vi "observacao.vi"() -> ()   [LabVIEW 2018, in "Shared_160.lvlib"] (continued)
                w2479 = u16 15 items=["Alarme", "Atencao", "Erro", "Ocupado", "PosSecund", "PosConj#3", "MovFoco", "MovCjto#3", "Mov#4", "Mov#3", "Mov#2", "EspLamp", "HE", "NE", "EspLampRepouso", "EspLampCalibra"] ("NomeStatus")
                w2480 = u16 14 items=["Alarme", "Atencao", "Erro", "Ocupado", "PosSecund", "PosConj#3", "MovFoco", "MovCjto#3", "Mov#4", "Mov#3", "Mov#2", "EspLamp", "HE", "NE", "EspLampRepouso", "EspLampCalibra"] ("NomeStatus")
                w2481 = u16 11 items=["Alarme", "Atencao", "Erro", "Ocupado", "PosSecund", "PosConj#3", "MovFoco", "MovCjto#3", "Mov#4", "Mov#3", "Mov#2", "EspLamp", "HE", "NE", "EspLampRepouso", "EspLampCalibra"] ("NomeStatus")
                # "Cassegrain"
                n1920 = event shown="[3] \"Sent_EspLampCass\": Value Change" {
                  selector: _ -> [_ _ _ _]
                  dyn-events: _ -> [_ _ _ _]
                  timeout: 10 -> [_ _ _ _]
                  event Timeout {
                    n1921 = event-data() -> ()  [unwired: 1 in, 2 out]
                  }
                  event "Ne": Value Change {
                    w2508 = u16 3 items=["ZERO", "AH", "DEC", "TUBO", "CUP"] ("Controlador")
                    n1922 = event-data() -> ()  [unwired: 1 in, 1 out]
                    n1923 = case shown="True" "Ne" {
                      tunnel: ["LAMP_NE" "LAMP_NE"] -> w2507
                      tunnel: ["DESLIGAR" "LIGAR"] -> w2506
                      frame False {
                      }
                      frame True {
                      }
                    }
                    n1924 = call "Monta Comando.vi"("Comando"=w2506, "Dispositivo"=w2507, "Controlador"=w2508) -> ()  [unwired: 2 in, 5 out]
                  }
                  event "He-Ar": Value Change {
                    w2516 = u16 3 items=["ZERO", "AH", "DEC", "TUBO", "CUP"] ("Controlador")
                    n1925 = event-data() -> ()  [unwired: 1 in, 1 out]
                    n1926 = case shown="False" "He-Ar" {
                      tunnel: ["LAMP_HE" "LAMP_HE"] -> w2515
                      tunnel: ["DESLIGAR" "LIGAR"] -> w2514
                      frame False {
                      }
                      frame True {
                      }
                    }
                    n1927 = call "Monta Comando.vi"("Comando"=w2514, "Dispositivo"=w2515, "Controlador"=w2516) -> ()  [unwired: 2 in, 5 out]
                  }
                  event "Sent_EspLampCass": Value Change {
                    w2524 = u16 3 items=["ZERO", "AH", "DEC", "TUBO", "CUP"] ("Controlador")
                    n1928 = event-data() -> ()  [unwired: 1 in, 1 out]
                    n1929 = property on="SlideEcass" class="Slide (strict)"("Visible"=TRUE) -> ()  [unwired: 2 in, 2 out]
                    n1930 = case shown="False" "Sent_EspLampCass" {
                      tunnel: ["ESP_LAMP" "ESP_LAMP"] -> w2523
                      tunnel: ["RECUAR" "AVANCAR"] -> w2522
                      frame False {
                      }
                      frame True {
                      }
                    }
                    n1931 = property on="stopEcass" class="Bool"("Visible"=FALSE) -> ()  [unwired: 2 in, 2 out]
                    n1932 = call "Monta Comando.vi"("Comando"=w2522, "Dispositivo"=w2523, "Controlador"=w2524) -> ()  [unwired: 2 in, 5 out]
                    "SlideEcass" <- u8 8 ("Slide")
                  }
                }
                n1933 = call "Bit Status TUBO.vi"("NomeStatus"=w2477) -> ("StatBit"=→"LedHe":bool)
                n1934 = call "Bit Status TUBO.vi"("NomeStatus"=w2478) -> ("StatBit"=→"LedNe":bool)
                n1935 = call "Bit Status TUBO.vi"("NomeStatus"=w2481) -> ("StatBit"=w2476:bool)
                n1936 = call "Bit Status TUBO.vi"("NomeStatus"=w2480) -> ("StatBit"=w2475:bool)
                n1937 = call "Bit Status TUBO.vi"("NomeStatus"=w2479) -> ("StatBit"=w2474:bool)
                n1938 = And(x=w2476, y=w2475) -> (x .and. y?=w2473:bool)
                "LedRep" <- w2473
                n1939 = And(x=w2476, y=w2474) -> (x .and. y?=w2472:bool)
                "LedCal" <- w2472
                n1940 = property on="SlideEcass" class="Slide (strict)"() -> ("Visible"=w2471:bool)  [unwired: 2 in, 2 out]
                n1941 = Or(x=w2473, y=w2472) -> (x .or. y?=w2483:bool)
                n1942 = Or(x=w2475, y=w2474) -> (x .or. y?=w2486:bool)
                n1943 = Not(x=w2476) -> (.not. x?=w2485:bool)
                n1944 = And(x=w2471, y=w2483) -> (x .and. y?=w2482:bool)
                n1945 = And(x=w2485, y=w2486) -> (x .and. y?=w2484:bool)
                n1946 = case shown="True" "stopEcass" {
                  frame False {
                  }
                  frame True {
                    w2503 = FALSE
                    w2502 = u8 0 ("Disabled")
                    w2501 = u16 3 items=["ZERO", "AH", "DEC", "TUBO", "CUP"] ("Controlador")
                    n1947 = call "Monta Comando.vi"("Comando"="DESLIGAR", "Dispositivo"="ESP_LAMP", "Controlador"=w2501) -> ()  [unwired: 2 in, 5 out]
                    n1948 = property on="Sent_EspLampCass" class="Bool (strict)"("Disabled"=w2502) -> ()  [unwired: 2 in, 2 out]
                    n1949 = property on="Ne" class="Bool (strict)"("Disabled"=w2502) -> ()  [unwired: 2 in, 2 out]
                    n1950 = property on="He-Ar" class="Bool (strict)"("Disabled"=w2502) -> ()  [unwired: 2 in, 2 out]
                    n1951 = property on="SlideEcass" class="Slide (strict)"("Visible"=w2503) -> ()  [unwired: 2 in, 2 out]
                    n1952 = property on="stopEcass" class="Bool"("Visible"=w2503) -> ()  [unwired: 2 in, 2 out]
                  }
                }
                n1953 = case shown="True" w2482 {
                  frame False {
                  }
                  frame True {
                    w2504 = u8 0 ("Disabled")
                    n1954 = property on="Sent_EspLampCass" class="Bool (strict)"("Disabled"=w2504) -> ()  [unwired: 2 in, 2 out]
                    n1955 = property on="He-Ar" class="Bool (strict)"("Disabled"=w2504) -> ()  [unwired: 2 in, 2 out]
                    n1956 = property on="Ne" class="Bool (strict)"("Disabled"=w2504) -> ()  [unwired: 2 in, 2 out]
                    n1957 = property on="SlideEcass" class="Slide (strict)"("Visible"=FALSE) -> ()  [unwired: 2 in, 2 out]
                  }
                }
                n1958 = case shown="True" w2484 {
                  frame False {
                  }
                  frame True {
                    w2488 = u8 2 ("Disabled")
                    n1959 = local read "SlideEcass"() -> (w2489:u8)
                    n1960 = property on="Sent_EspLampCass" class="Bool (strict)"("Disabled"=w2488) -> ()  [unwired: 2 in, 2 out]
                    n1961 = property on="Ne" class="Bool (strict)"("Disabled"=w2488) -> ()  [unwired: 2 in, 2 out]
                    n1962 = property on="He-Ar" class="Bool (strict)"("Disabled"=w2488) -> ()  [unwired: 2 in, 2 out]
                    n1963 = Add(x=w2489, y=u8 4) -> (x+y=w2491:u8)
                    n1964 = Greater Or Equal?(x=w2491, y=u8 100 ("x")) -> (x >= y?=w2492:bool)
                    n1965 = case shown="True" w2492 {
                      selector: w2492 -> [_ w2496]
                      tunnel: w2491 -> [w2495 _]
                      frame False {
                        n1966 = local write "SlideEcass"(w2495) -> ()
                        n1967 = property on="SlideEcass" class="Slide (strict)"("Fill Color"=u32 16750950 ("color(black)")) -> ()  [unwired: 2 in, 2 out]
                      }
                      frame True {
                        n1968 = local write "SlideEcass"(u8 92 ("Slide")) -> ()
                        n1969 = property on="stopEcass" class="Bool"("Visible"=w2496) -> ()  [unwired: 2 in, 2 out]
                        n1970 = property on="SlideEcass" class="Slide (strict)"("Fill Color"=u32 16724787 ("color(black)")) -> ()  [unwired: 2 in, 2 out]
                      }
                    }
                  }
                }
              }
              frame "Eucalyp." {
                # "Eucalyptus"
              }
              frame "Cam 1" {
              }
              frame "Cam 2" {
                # "Cam 2"
              }
              frame "Cam IV." {
                # "Cam IV"
              }
              frame "Polarim." {
                # "Polarimetro"
              }
              frame "Fotrap" {
                # "Fotrap"
              }
              frame "Coude", Default {
                # "COUDE"
                n1971 = stacked-sequence {
                  frame #0 {
                    w2535 = u16 5 items=["Alarme", "Atencao", "Erro", "Ocupado", "Stop#3", "Cass#3", "MovFoco", "PosSecund", "Mov#2", "Mov#3", "Mov#4", "EspLamp", "HE", "NE", "EspLampRepouso", "EspLampCalibra"] ("NomeStatus")
                    w2534 = u16 7 items=["Alarme", "Atencao", "Erro", "Ocupado", "Stop#3", "Cass#3", "MovFoco", "PosSecund", "Mov#2", "Mov#3", "Mov#4", "EspLamp", "HE", "NE", "EspLampRepouso", "EspLampCalibra"] ("NomeStatus")
                    n1972 = local read "EspAtual"() -> (w2537:string)
                    n1973 = case shown="\"A\"" w2537 {
                      frame "X", Default {
                        w2538 = FALSE
                        n1974 = local write "ledVisivel"(w2538) -> ()
                        n1975 = local write "ledAzul"(w2538) -> ()
                        n1976 = local write "ledVermelho"(w2538) -> ()
                      }
                      frame "M" {
                        w2539 = FALSE
                        n1977 = local write "ledAzul"(w2539) -> ()
                        n1978 = local write "ledVermelho"(w2539) -> ()
                        n1979 = local write "ledVisivel"(w2539) -> ()
                      }
                      frame "A" {
                        # "Espelho A --> Azul\nEspelho B --> Visível\nEspelho C --> Vermelho"
                        n1980 = local write "ledVermelho"(FALSE) -> ()
                        n1981 = local write "ledVisivel"(FALSE) -> ()
                        n1982 = local write "ledAzul"(TRUE) -> ()
                      }
                      frame "B" {
                        # "Espelho A --> Azul\nEspelho B --> Visível\nEspelho C --> Vermelho"
                        n1983 = local write "ledVermelho"(FALSE) -> ()
                        n1984 = local write "ledVisivel"(TRUE) -> ()
                        n1985 = local write "ledAzul"(FALSE) -> ()
                      }
                      frame "C" {
                        # "Espelho A --> Azul\nEspelho B --> Visível\nEspelho C --> Vermelho"
                        n1986 = local write "ledVermelho"(TRUE) -> ()
                        n1987 = local write "ledVisivel"(FALSE) -> ()
                        n1988 = local write "ledAzul"(FALSE) -> ()
                      }
                    }
                    n1989 = call "Bit Status TUBO.vi"("NomeStatus"=w2535) -> ("StatBit"=→"Cjto_3":bool)
                    n1990 = call "Bit Status TUBO.vi"("NomeStatus"=w2534) -> ("StatBit"=→"PosSecundario":bool)
                  }
                  frame #1 {
                    w2559 = u16 5 items=["Alarme", "Atencao", "Erro", "Ocupado", "Stop#3", "Cass#3", "MovFoco", "PosSecund", "Mov#2", "Mov#3", "Mov#4", "EspLamp", "HE", "NE", "EspLampRepouso", "EspLampCalibra"] ("NomeStatus")
                    w2564 = u16 8 items=["Alarme", "Atencao", "Erro", "Ocupado", "Stop#3", "Cass#3", "MovFoco", "PosSecund", "Mov#2", "Mov#3", "Mov#4", "EspLamp", "HE", "NE", "EspLampRepouso", "EspLampCalibra"] ("NomeStatus")
                    w2565 = u16 9 items=["Alarme", "Atencao", "Erro", "Ocupado", "Stop#3", "Cass#3", "MovFoco", "PosSecund", "Mov#2", "Mov#3", "Mov#4", "EspLamp", "HE", "NE", "EspLampRepouso", "EspLampCalibra"] ("NomeStatus")
                    w2566 = u16 10 items=["Alarme", "Atencao", "Erro", "Ocupado", "Stop#3", "Cass#3", "MovFoco", "PosSecund", "Mov#2", "Mov#3", "Mov#4", "EspLamp", "HE", "NE", "EspLampRepouso", "EspLampCalibra"] ("NomeStatus")
                    w2577 = u16 4 items=["Alarme", "Atencao", "Erro", "Ocupado", "Stop#3", "Cass#3", "MovFoco", "PosSecund", "Mov#2", "Mov#3", "Mov#4", "EspLamp", "HE", "NE", "EspLampRepouso", "EspLampCalibra"] ("NomeStatus")
                    w2578 = u16 3 items=["Alarme", "Atencao", "Erro", "Ocupado", "Stop#3", "Cass#3", "MovFoco", "PosSecund", "Mov#2", "Mov#3", "Mov#4", "EspLamp", "HE", "NE", "EspLampRepouso", "EspLampCalibra"] ("NomeStatus")
                    # "CJTO#3 EM \nMOVIMENTO"
                    n1991 = local read "PosSecundario"() -> (w2557:bool)
                    n1992 = call "Bit Status TUBO.vi"("NomeStatus"=w2559) -> ("StatBit"=w2556:bool)
                    n1993 = call "Bit Status TUBO.vi"("NomeStatus"=w2577) -> ("StatBit"=w2555:bool)
                    n1994 = call "Bit Status TUBO.vi"("NomeStatus"=w2578) -> ("StatBit"=w2553:bool)
                    n1995 = call "Bit Status TUBO.vi"("NomeStatus"=w2564) -> ("StatBit"=w2570:bool)
                    "#2" <- w2570
                    n1996 = call "Bit Status TUBO.vi"("NomeStatus"=w2565) -> ("StatBit"=w2569:bool)
                    "#3" <- w2569
                    n1997 = call "Bit Status TUBO.vi"("NomeStatus"=w2566) -> ("StatBit"=w2568:bool)
                    "#4" <- w2568
                    n1998 = Not Equal?(x=w2557, y=w2556) -> (x != y?=w2558:bool)
                    n1999 = Not(x=w2555) -> (.not. x?=w2551:bool)
                    n2000 = And(x=w2558, y=w2555) -> (x .and. y?=w2552:bool)
                    n2001 = Compound Arithmetic op=OR(w2570, w2569, w2568) -> (w2567:bool)
                    n2002 = Compound Arithmetic op=OR(w2552, w2551, w2553) -> (w2554:bool)
                    n2003 = property on="Cjto_3" class="Bool (strict)"("Blinking"=w2552) -> ()  [unwired: 2 in, 2 out]
                    n2004 = property on="PosSecundario" class="Bool (strict)"("Blinking"=w2552) -> ()  [unwired: 2 in, 2 out]
                    n2005 = case shown="True" w2554 {
                      tunnel: [T6."Page Enabled" ("Page Enabled State") T6."Page Disabled" ("Page Enabled State")] -> w2549
                      tunnel: [u8 0 ("Disabled") u8 2 ("Disabled")] -> w2563
                      frame False {
                      }
                      frame True {
                      }
                    }
                    n2006 = property on="MENSAGEM" class="Str"("Visible"=w2551, "Blinking"=w2551) -> ()  [unwired: 2 in, 2 out]
                    n2007 = case shown="True" w2567 {
                      tunnel: w2563 -> [w2582 _]
                      tunnel: [w2582 u8 2 ("Disabled")] -> w2562
                      tunnel: [FALSE TRUE] -> w2561
                      tunnel: [FALSE ("Blinking") TRUE ("Blinking")] -> w2560
                      frame False {
                        n2008 = local write "MENSAGEM 2"("EM MOVIMENTO" ("MENSAGEM 2")) -> ()
                      }
                      frame True {
                        n2009 = local read "EndTime"() -> (w2591:u32)
                        n2010 = Tick Count (ms)() -> (millisecond timer value=w2590:u32)
                        n2011 = Subtract(x=w2591, y=w2590) -> (x-y=w2589:u32)
                        n2012 = Divide(x=w2589, y=u32 1000) -> (x/y=w2586:dbl)
                        n2013 = To Unsigned Long Integer(number=w2586) -> (unsigned 32bit integer=w2587:u32)
                        n2014 = Number To Decimal String(number=w2587) -> (decimal integer string=w2584:string)  [unwired: 1 in]
                        n2015 = Concatenate Strings("EM MOVIMENTO " ("MENSAGEM 2"), w2584) -> (w2585:string)
                        n2016 = local write "MENSAGEM 2"(w2585) -> ()
                      }
                    }
                    n2017 = property on="Setup, Pointing & Guiding" class="TabCtl (strict)"() -> ("Pages"=w2550:refnum<vi>[])  [unwired: 2 in, 2 out]
                    n2018 = Index Array(array=w2550, index=4) -> (element=w2573:refnum<vi>)
                    n2019 = Index Array(array=w2550, index=5) -> (element=w2576:refnum<vi>)
                    n2020 = property class="Page"(reference=w2573, "Page Enabled State"=w2549) -> ()  [unwired: 1 in, 2 out]
                    n2021 = property class="Page"(reference=w2576, "Page Enabled State"=w2549) -> ()  [unwired: 1 in, 2 out]
                    n2022 = case shown="False" w2557 {
                      tunnel: [u8 0 ("Disabled") w2597] -> w2572
                      tunnel: w2562 -> [w2595 _]
                      tunnel: [w2595 w2597] -> w2571
                      frame False {
                        # "COUDE"
                      }
                      frame True {
                        w2597 = u8 2 ("Disabled")
                        # "CASS"
                      }
                    }
                    n2023 = property on="MENSAGEM 2" class="Str"("Visible"=w2561, "Blinking"=w2560) -> ()  [unwired: 2 in, 2 out]
                    n2024 = property on="ledAzul" class="Bool (strict)"("Disabled"=w2572) -> ()  [unwired: 2 in, 2 out]
                    n2025 = property on="ledVisivel" class="Bool (strict)"("Disabled"=w2572) -> ()  [unwired: 2 in, 2 out]
                    n2026 = property on="ledVermelho" class="Bool (strict)"("Disabled"=w2572) -> ()  [unwired: 2 in, 2 out]
                    n2027 = property on="Radio Buttons" class="RadioBtnsControl (strict)"("Disabled"=w2572) -> ()  [unwired: 2 in, 2 out]
                    n2028 = property on="#2" class="Bool (strict)"("Disabled"=w2572) -> ()  [unwired: 2 in, 2 out]
                    n2029 = property on="#3" class="Bool (strict)"("Disabled"=w2572) -> ()  [unwired: 2 in, 2 out]
                    n2030 = property on="#4" class="Bool (strict)"("Disabled"=w2572) -> ()  [unwired: 2 in, 2 out]
                    n2031 = property on="Go_Coudé" class="Bool"("Disabled"=w2571) -> ()  [unwired: 2 in, 2 out]
                  }
                  frame #2 {
                    n2032 = case shown="True" "Go_Coudé" {
                      frame False {
                        w2603 = u16 2 items=["Alarme", "Atencao", "Erro", "Ocupado", "Stop#3", "Cass#3", "MovFoco", "PosSecund", "Mov#2", "Mov#3", "Mov#4", "EspLamp", "HE", "NE", "EspLampRepouso", "EspLampCalibra"] ("NomeStatus")
                        w2604 = u16 3 items=["Alarme", "Atencao", "Erro", "Ocupado", "Stop#3", "Cass#3", "MovFoco", "PosSecund", "Mov#2", "Mov#3", "Mov#4", "EspLamp", "HE", "NE", "EspLampRepouso", "EspLampCalibra"] ("NomeStatus")
                        # "TRATA ERROS DO CONTROLADOR"
                        n2033 = call "Bit Status TUBO.vi"("NomeStatus"=w2603) -> ("StatBit"=w2606:bool)
                        n2034 = call "Bit Status TUBO.vi"("NomeStatus"=w2604) -> ("StatBit"=w2608:bool)
                        n2035 = Not(x=w2608) -> (.not. x?=w2607:bool)
                        n2036 = And(x=w2606, y=w2607) -> (x .and. y?=w2605:bool)
                        n2037 = case shown="True" w2605 {
                          frame False {
                          }
                          frame True {
                            w2611 = u16 3 items=["ZERO", "AH", "DEC", "TUBO", "CUP"] ("Controlador")
                            n2038 = call "Monta Comando.vi"("Comando"="ERROS", "Dispositivo"="PROG" ("Comando"), "Controlador"=w2611) -> ()  [unwired: 2 in, 5 out]
                          }
                        }
                      }
                      frame True {
                        w2612 = u16 3 items=["ZERO", "AH", "DEC", "TUBO", "CUP"] ("Controlador")
                        # "Enviar comando de \nmudar Espelho ABC"
                        n2039 = local read "EspAtual"() -> (w2618:string)
                        n2040 = case shown="\"Visível\"" "Radio Buttons" {
                          tunnel: ["C" ("Comando") "A" ("Comando") "B" ("Comando")] -> w2613
                          tunnel: w2618 -> [w2621 w2627 w2632]
                          tunnel: [w2620 w2626 w2633] -> w2615
                          frame "Vermelho" {
                            n2041 = case shown="\"A\"" w2621 {
                              tunnel: [u32 0 u32 60000 u32 35000] -> w2620
                              frame "C", Default {
                              }
                              frame "B" {
                              }
                              frame "A" {
                              }
                            }
                          }
                          frame "Azul", Default {
                            n2042 = case shown="\"C\"" w2627 {
                              tunnel: [u32 0 u32 35000 u32 60000] -> w2626
                              frame "A", Default {
                              }
                              frame "B" {
                              }
                              frame "C" {
                              }
                            }
                          }
                          frame "Visível" {
                            n2043 = case shown="\"C\"" w2632 {
                              tunnel: [u32 0 u32 60000 u32 35000] -> w2633
                              frame "B", Default {
                              }
                              frame "A" {
                              }
                              frame "C" {
                              }
                            }
                          }
                        }
                        n2044 = Tick Count (ms)() -> (millisecond timer value=w2617:u32)
                        n2045 = Add(x=w2617, y=w2615) -> (x+y=→"EndTime":u32)
                        n2046 = call "Monta Comando.vi"("Comando"=w2613, "Dispositivo"="ESPELHO" ("Comando"), "Controlador"=w2612) -> ()  [unwired: 2 in, 5 out]
                      }
                    }
                  }
                  frame #3 {
                    w2644 = 360.0
                    w2649 = 6.283185307179586
                    n2047 = global read "Global_Telescopio.vi" "guide_ang"() -> (w2659:string)
                    n2048 = global read "Global_Telescopio.vi" "guide_nor"() -> (w2660:string)
                    n2049 = global read "Global_Telescopio.vi" "AH_now"() -> (w2656:dbl)
                    n2050 = global read "Global_Telescopio.vi" "delta_now"() -> (w2657:dbl)
                    n2051 = Add(x=w2656, y=w2657) -> (x+y=w2648:dbl)
                    n2052 = Fract/Exp String To Number(string=w2659) -> (number=w2655:dbl)  [unwired: 3 in, 1 out]
                    n2053 = Fract/Exp String To Number(string=w2660) -> (number=w2658:dbl)  [unwired: 3 in, 1 out]
                    n2054 = Quotient & Remainder(x=w2648, y=w2649) -> (x-y*floor(x/y)=w2651:dbl)  [unwired: 1 out]
                    n2055 = Add(x=w2655, y=w2658) -> (x+y=w2640:dbl)
                    n2056 = Less Than 0?(x=w2651) -> (x < 0?=w2653:bool)
                    n2057 = case shown="True" w2653 {
                      tunnel: w2651 -> [w2661 w2664]
                      tunnel: [w2661 w2662] -> w2650
                      tunnel: w2649 -> [_ w2663]
                      frame False {
                      }
                      frame True {
                        n2058 = Add(x=w2664, y=w2663) -> (x+y=w2662:dbl)
                      }
                    }
                    n2059 = Add(x=124.0, y=w2640) -> (x+y=w2639:dbl)
                    n2060 = Multiply(x=w2650, y=57.29577951 ("x*y")) -> (x*y=w2647:dbl)
                    n2061 = Subtract(x=98.2, y=w2647) -> (x-y=w2646:dbl)
                    n2062 = Add(x=w2639, y=w2646) -> (x+y=w2643:dbl)
                    n2063 = Quotient & Remainder(x=w2643, y=w2644) -> (floor(x/y)=w2645:dbl)  [unwired: 1 out]
                    n2064 = Multiply(x=w2645, y=w2644) -> (x*y=w2642:dbl)
                    n2065 = Subtract(x=w2643, y=w2642) -> (x-y=→"Ang. Fenda":dbl)
                  }
                  frame #4 {
                    # "90"
                    # "270"
                    # "180"
                    # "0"
                    n2066 = event shown="[7] \"Go Angulo de Difração\": Value Change" {
                      selector: _ -> [_ _ _ _ _ _ _ _ _ _ _]
                      dyn-events: _ -> [_ _ _ _ _ _ _ _ _ _ _]
                      timeout: 10 -> [_ _ _ _ _ _ _ _ _ _ _]
                      event Timeout {
                        n2067 = event-data() -> ()  [unwired: 1 in, 2 out]
                        n2068 = stacked-sequence {
                          frame #0 {
                            n2069 = local read "parou 3"() -> (w2666:bool)
                            n2070 = case shown="True" w2666 {
                              frame False {
                              }
                              frame True {
                                n2071 = call "InstrumentControl.vi"("Input Message"="COUDE REDE POSICAO") -> ("Output Message"=w2669:string)  [unwired: 9 in, 1 out]
                                "Output Message" <- w2669
                                n2072 = Decimal String To Number(string=w2669) -> (number=w2668:i32)  [unwired: 2 in, 1 out]
                                n2073 = while {
                                shift-right: [w2672] -> w2667
                                shift-left: _ -> [w2676]
                                tunnel: w2668 -> [w2672]
                                stop <- TRUE stop-if-true
                                n2074 = Subtract(x=w2676, y=w2672) -> (x-y=w2675:i32)
                                n2075 = Absolute Value(x=w2675) -> (abs(x)=w2674:i32)
                                n2076 = Greater Or Equal?(x=w2674, y=1) -> (x >= y?=→"parou 3":bool)
                                }
                                "Posição Rede" <- w2667
                              }
                            }
                          }
                          frame #1 {
                            n2077 = local read "parou"() -> (w2679:bool)
                            n2078 = local read "parou 2"() -> (w2678:bool)
                            n2079 = case shown="True" w2678 {
                              frame False {
                              }
                              frame True {
                                # "Cada volta -> 10mm\nCada volta -> 4000counts\n1 count = 0,0025mm"
                                n2080 = call "InstrumentControl.vi"("Input Message"="COUDE ESPELHO POSICAO") -> ("Output Message"=w2686:string)  [unwired: 9 in, 1 out]
                                n2081 = Fract/Exp String To Number(string=w2686) -> (number=w2685:dbl)  [unwired: 3 in, 1 out]
                                n2082 = while {
                                shift-right: [w2698] -> w2681
                                shift-left: _ -> [w2699]
                                tunnel: w2685 -> [w2698]
                                tunnel: [w2694] -> w2680
                                stop <- TRUE stop-if-true
                                n2083 = Subtract(x=w2699, y=w2698) -> (x-y=w2697:dbl)
                                n2084 = Absolute Value(x=w2697) -> (abs(x)=w2696:dbl)
                                n2085 = Greater Or Equal?(x=w2696, y=0.02) -> (x >= y?=w2694:bool)
                                "parou 2" <- w2694
                                }
                                "Posição Espelho" <- w2681
                                n2086 = case shown="False" w2680 {
                                frame False {
                                n2087 = call "InstrumentControl.vi"("Input Message"="COUDE SERIAL CHAVEAR OFF") -> ()  [unwired: 9 in, 2 out]
                                }
                                frame True {
                                }
                                }
                                n2088 = Absolute Value(x=w2681) -> (abs(x)=w2682:dbl)
                                n2089 = Less Or Equal?(x=w2682, y=0.5) -> (x <= y?=w2684:bool)
                                n2090 = case shown="False" w2684 {
                                tunnel: w2682 -> [w2691 _]
                                frame False {
                                n2091 = Greater Or Equal?(x=w2691, y=34.5) -> (x >= y?=w2689:bool)
                                n2092 = case shown="True" w2689 {
                                frame False {
                                }
                                frame True {
                                n2093 = local write "Boolean"(TRUE ("Boolean")) -> ()
                                }
                                }
                                }
                                frame True {
                                n2094 = local write "Boolean"(FALSE ("Boolean")) -> ()
                                }
                                }
                              }
                            }
                            n2095 = case shown="True" w2679 {
                              frame False {
                              }
                              frame True {
                                n2096 = call "InstrumentControl.vi"("Input Message"="COUDE FENDA POSICAO") -> ("Output Message"=w2706:string)  [unwired: 9 in, 1 out]
                                n2097 = Fract/Exp String To Number(string=w2706) -> (number=w2705:dbl)  [unwired: 3 in, 1 out]
                                n2098 = Multiply(x=w2705, y=1000.0) -> (x*y=w2703:dbl)
                                n2099 = while {
                                shift-right: [w2713] -> w2702
                                shift-left: _ -> [w2714]
                                tunnel: w2703 -> [w2713]
                                tunnel: [w2709] -> w2701
                                stop <- TRUE stop-if-true
                                n2100 = Subtract(x=w2714, y=w2713) -> (x-y=w2712:dbl)
                                n2101 = Absolute Value(x=w2712) -> (abs(x)=w2711:dbl)
                                n2102 = Greater Or Equal?(x=w2711, y=1.0) -> (x >= y?=w2709:bool)
                                "parou" <- w2709
                                }
                                "Largura da Fenda 2" <- w2702
                                n2103 = case shown="False" w2701 {
                                frame False {
                                n2104 = call "InstrumentControl.vi"("Input Message"="COUDE SERIAL CHAVEAR OFF") -> ()  [unwired: 9 in, 2 out]
                                }
                                frame True {
                                }
                                }
                              }
                            }
                          }
                        }
                      }
                      event "Cathode": Value Change {
                        n2105 = event-data() -> ("NewVal"=w2716:bool)  [unwired: 1 in, 4 out]
                        n2106 = case shown="True" w2716 {
                          frame False {
                          }
                          frame True {
                            n2107 = flat-sequence {
                              frame #0 {
                                w2718 = FALSE ("NeAr")
                                n2108 = local write "Neon"(w2718) -> ()
                                n2109 = local write "Incand"(w2718) -> ()
                                n2110 = local write "Position"("Moving" ("Prisma Position")) -> ()
                                n2111 = call "Comando_Quick_Silver.vi"("COMANDO COMPLETO"="COUDE PRISMA MOVER 0" ("Input Message")) -> ()  [unwired: 2 in, 3 out]
                                n2112 = local write "IronArc"(w2718) -> ()
                              }
                              frame #1 {
                                n2113 = Wait (ms)(milliseconds to wait=u32 50) -> ()  [unwired: 1 out]
                              }
                              frame #2 {
                                n2114 = local write "Position"("Cathode" ("Prisma Position")) -> ()
                              }
                            }
                          }
                        }
                      }
                      event "Neon": Value Change {
                        n2115 = event-data() -> ("NewVal"=w2722:bool)  [unwired: 1 in, 4 out]
                        n2116 = case shown="True" w2722 {
                          frame False {
                          }
                          frame True {
                            n2117 = flat-sequence {
                              frame #0 {
                                w2724 = FALSE ("ThAr")
                                n2118 = local write "Cathode"(w2724) -> ()
                                n2119 = local write "Incand"(w2724) -> ()
                                n2120 = local write "Position"("Moving" ("Prisma Position")) -> ()
                                n2121 = call "Comando_Quick_Silver.vi"("COMANDO COMPLETO"="COUDE PRISMA MOVER 180" ("Input Message")) -> ()  [unwired: 2 in, 3 out]
                                n2122 = local write "IronArc"(w2724) -> ()
                              }
                              frame #1 {
                                n2123 = Wait (ms)(milliseconds to wait=u32 50) -> ()  [unwired: 1 out]
                              }
                              frame #2 {
                                n2124 = local write "Position"("Neon" ("Prisma Position")) -> ()
                              }
                            }
                          }
                        }
                      }
                      event "Incand": Value Change {
                        n2125 = event-data() -> ("NewVal"=w2728:bool)  [unwired: 1 in, 4 out]
                        n2126 = case shown="True" w2728 {
                          frame False {
                          }
                          frame True {
                            n2127 = flat-sequence {
                              frame #0 {
                                w2730 = FALSE ("ThAr")
                                n2128 = local write "Cathode"(w2730) -> ()
                                n2129 = local write "Neon"(w2730) -> ()
                                n2130 = local write "Position"("Moving" ("Prisma Position")) -> ()
                                n2131 = call "Comando_Quick_Silver.vi"("COMANDO COMPLETO"="COUDE PRISMA MOVER 270 " ("Input Message")) -> ()  [unwired: 2 in, 3 out]
                                n2132 = local write "IronArc"(w2730) -> ()
                              }
                              frame #1 {
                                n2133 = Wait (ms)(milliseconds to wait=u32 50) -> ()  [unwired: 1 out]
                              }
                              frame #2 {
                                n2134 = local write "Position"("Incand" ("Prisma Position")) -> ()
                              }
                            }
                          }
                        }
                      }
                      event Value Change {
                        n2135 = event-data() -> ("NewVal"=w2734:T4)  [unwired: 1 in, 4 out]
                        n2136 = case shown="True" w2734 {
                          frame False {
                          }
                          frame True {
                            n2137 = call "InstrumentControl.vi"("Input Message"="COUDE FENDA INICIAR") -> ()  [unwired: 9 in, 2 out]
                          }
                        }
                      }
                      event Value Change {
                        n2138 = event-data() -> ("NewVal"=w2736:T4)  [unwired: 1 in, 4 out]
                        n2139 = case shown="True" w2736 {
                          frame False {
                          }
                          frame True {
                            n2140 = call "Comando_Quick_Silver.vi"("COMANDO COMPLETO"="COUDE ESPELHO INICIAR" ("Input Message")) -> ()  [unwired: 2 in, 3 out]
                          }
                        }
                      }
                      event Value Change {
                        n2141 = event-data() -> ("NewVal"=w2738:T4)  [unwired: 1 in, 4 out]
                        n2142 = case shown="True" w2738 {
                          frame False {
                          }
                          frame True {
                            n2143 = call "InstrumentControl.vi"("Input Message"="COUDE PRISMA INICIAR") -> ()  [unwired: 9 in, 2 out]
                          }
                        }
                      }
                      event "Go Angulo de Difração": Value Change {
                        n2144 = event-data() -> ("NewVal"=w2740:bool)  [unwired: 1 in, 4 out]
                        n2145 = case shown="True" w2740 {
                          frame False {
                          }
                          frame True {
                            # "Envia comando para rede de difração"
                            n2146 = Number To Decimal String(number="Angulo da rede de difração") -> (decimal integer string=w2742:string)  [unwired: 1 in]
                            n2147 = Concatenate Strings("COUDE REDE MOVER ", w2742) -> (w2745:string)
                            n2148 = call "InstrumentControl.vi"("Input Message"=w2745) -> ()  [unwired: 9 in, 2 out]
                            n2149 = local write "parou 3"(TRUE ("parou 3")) -> ()
                          }
                        }
                      }
                      event "Go Largura da Fenda": Value Change {
                        n2150 = event-data() -> ("NewVal"=w2746:bool)  [unwired: 1 in, 4 out]
                        n2151 = case shown="True" w2746 {
                          frame False {
                          }
                          frame True {
                            n2152 = call "InstrumentControl.vi"("Input Message"="COUDE SERIAL CHAVEAR ON") -> ("error out"=w2748:errorcluster)  [unwired: 9 in, 1 out]
                            n2153 = Divide(x="Largura da Fenda", y=1000.0) -> (x/y=w2756:dbl)
                            n2154 = Number To Fractional String(use system decimal point (T)=FALSE, number=w2756, precision (6)=i16 6) -> (F-format string=w2750:string)  [unwired: 1 in]
                            n2155 = Concatenate Strings("COUDE FENDA MOVER ", w2750) -> (w2752:string)
                            n2156 = local write "parou"(TRUE ("parou")) -> ()
                            n2157 = call "InstrumentControl.vi"("error"=w2748, "Input Message"=w2752) -> ()  [unwired: 8 in, 2 out]
                          }
                        }
                      }
                      event "Prisma das Lâmpadas": Value Change {
                        n2158 = event-data() -> ("NewVal"=w2767:bool)  [unwired: 1 in, 4 out]
                        n2159 = case shown="False" w2767 {
                          tunnel: [0.0 ("y") 35.0 ("y")] -> w2765
                          frame False {
                            n2160 = local write "Boolean"(TRUE ("Boolean")) -> ()
                          }
                          frame True {
                            n2161 = local write "Boolean"(FALSE ("Boolean 2")) -> ()
                          }
                        }
                        n2162 = local write "parou 2"(TRUE ("parou 2")) -> ()
                        n2163 = call "InstrumentControl.vi"("Input Message"="COUDE SERIAL CHAVEAR ON") -> ("error out"=w2759:errorcluster)  [unwired: 9 in, 1 out]
                        n2164 = Number To Fractional String(use system decimal point (T)=FALSE, number=w2765, precision (6)=i16 6) -> (F-format string=w2760:string)  [unwired: 1 in]
                        n2165 = Concatenate Strings("COUDE ESPELHO MOVER ", w2760) -> (w2762:string)
                        n2166 = call "InstrumentControl.vi"("error"=w2759, "Input Message"=w2762) -> ()  [unwired: 8 in, 2 out]
                      }
                      event "IronArc": Value Change {
                        n2167 = event-data() -> ("NewVal"=w2772:bool)  [unwired: 1 in, 4 out]
                        n2168 = case shown="True" w2772 {
                          frame False {
                          }
                          frame True {
                            n2169 = flat-sequence {
                              frame #0 {
                                w2774 = FALSE ("ThAr")
                                n2170 = local write "Cathode"(w2774) -> ()
                                n2171 = local write "Neon"(w2774) -> ()
                                n2172 = call "Comando_Quick_Silver.vi"("COMANDO COMPLETO"="COUDE PRISMA MOVER 90 " ("Input Message")) -> ()  [unwired: 2 in, 3 out]
                                n2173 = local write "Position"("Moving" ("Prisma Position")) -> ()
                                n2174 = local write "Incand"(w2774) -> ()
                              }
                              frame #1 {
                                n2175 = Wait (ms)(milliseconds to wait=u32 50) -> ()  [unwired: 1 out]
                              }
                              frame #2 {
                                n2176 = local write "Position"("IronArc" ("Prisma Position")) -> ()
                              }
                            }
                          }
                        }
                      }
                    }
                  }
                }
              }
            }
          }
          frame "FOCUS" {
            w2812 = cluster{u32, u32}[] [] ("Colors [4]")
            w2813 = cluster{u32, u32}[] [] ("Colors [4]")
            # "ATUALIZA FOCO COM VALORES\nPUBLICADOS PELO FOCUSER160"
            # "dark(0)/bright(1)\n green"
            # "red(0)/greem(1)"
            # "ZeroMQ"
            # "T:  0x54      84\nC: 0x43       51\nS:  0x53      83\nP:  0x50      80\nD:  0x44      52\nClientId= 350"
            n2177 = global read "Global_Telescopio.vi" "queueSUB"() -> (w2809:refnum<queue>)
            n2178 = global read "Global_Telescopio.vi" "Focuser160"() -> (w2805:T11)
            n2179 = Get Queue Status(queue=w2809) -> (queue out=w2806:refnum<queue>, # elements in queue=w2808:i32)  [unwired: 2 in, 6 out]
            n2180 = Greater Than 0?(x=w2808) -> (x > 0?=w2807:bool)
            n2181 = case shown="True" w2807 {
              tunnel: w2806 -> [_ w2843]
              tunnel: w2805 -> [w2834 w2841]
              tunnel: [w2834 w2840] -> w2804
              frame False {
              }
              frame True {
                n2182 = Flush Queue(queue=w2843) -> (remaining elements=w2837:string[], error out=w2842:errorcluster)  [unwired: 1 in, 1 out]
                n2183 = Array Size(array=w2837) -> (size(s)=w2839:i32)
                "size(s)" <- w2839
                n2184 = Decrement(x=w2839) -> (x-1=w2838:i32)
                n2185 = Index Array(array=w2837, index=w2838) -> (element=w2836:string)
                "element" <- w2836
                n2186 = call "Focuser JSON to cluster.vi"("JSON status"=w2836) -> ("Focuser160"=w2835:T11)  [unwired: 10 in]
                n2187 = Select(t=w2841, s=w2842, f=w2835) -> (s? t:f=w2840:T11)
                n2188 = global write "Global_Telescopio.vi" "Focuser160"(w2840) -> ()
              }
            }
            n2189 = Unbundle By Name(w2804) -> ("alarm"=→"focuAlarm":bool, "cmd"=w2802:T12, "connected"=w2801:bool, "maxSpeed"=w2800:dbl, "position"=→"Foco":dbl, "error"=w2795:string, "homing"=→"focusHoming":bool, "initialized"=→"focusInitialized":bool, "isMoving"=→"focusMoving":bool)  [unwired: 1 out]
            "focusConnected" <- w2801
            n2190 = Unbundle By Name(w2802) -> ("clientId"=w2825:dbl)
            n2191 = Search and Replace String(replace all?=TRUE ("replace all? (F)"), input string=w2795, search string="\"") -> (result string=w2792:string)  [unwired: 5 in, 3 out]
            n2192 = Select(t=w2813, s=w2801, f=w2812) -> (s? t:f=w2810:cluster{u32, u32}[])
            n2193 = Select(t=w2813, s=w2801, f=w2812) -> (s? t:f=w2811:cluster{u32, u32}[])
            n2194 = property on="focusInitialized" class="Bool (strict)"("Colors [4]"=w2810) -> ()  [unwired: 2 in, 2 out]
            n2195 = property on="focuAlarm" class="Bool (strict)"("Colors [4]"=w2811) -> ()  [unwired: 2 in, 2 out]
            n2196 = case shown="True" "SetDefaultFocus" {
              frame False {
              }
              frame True {
                n2197 = global read "Global_Telescopio.vi" "Foco Instrumento"() -> (w2882:string)
                n2198 = Fract/Exp String To Number(string=w2882) -> (number=w2881:dbl)  [unwired: 3 in, 1 out]
                n2199 = local write "Setpoint"(w2881) -> ()
              }
            }
            n2200 = Empty String/Path?(string/path=w2792) -> (empty?=w2829:bool)
            n2201 = To Unsigned Word Integer(number=w2800) -> (unsigned 16bit integer=w2824:u16)
            n2202 = Not Equal?(x=350.0, y=w2825) -> (x != y?=w2786:bool)
            n2203 = Not Equal To 0?(x=w2825) -> (x != 0?=w2785:bool)
            n2204 = Not(x=w2801) -> (.not. x?=w2783:bool)
            n2205 = Number To Decimal String(number=w2824) -> (decimal integer string=w2822:string)  [unwired: 1 in]
            n2206 = And(x=w2786, y=w2785) -> (x .and. y?=w2787:bool)
            n2207 = Or(x=w2787, y=w2783) -> (x .or. y?=w2784:bool)
            n2208 = Multiply(x=w2800, y="Velocity") -> (x*y=w2780:dbl)
            n2209 = Concatenate Strings("(max = " ("string"), w2822, " u/s)" ("string")) -> (w2816:string)
            n2210 = Select(t="            Focus Status", s=w2829, f=w2792) -> (s? t:f=→"focusStatus":string)
            n2211 = Divide(x=w2780, y=100.0) -> (x/y=w2778:dbl)
            n2212 = Select(t=T5."Disabled and Grayed Out" ("Disabled"), s=w2784, f=T5."Enabled" ("Disabled")) -> (s? t:f=w2788:T5)
            n2213 = property on="Velocity" class="Slide (strict)"("Caption.Text"=w2816) -> ()  [unwired: 2 in, 2 out]
            n2214 = property on="focusGo" class="Bool"("Disabled"=w2788) -> ()  [unwired: 2 in, 2 out]
            n2215 = property on="focusHome" class="Bool"("DisabledEnum"=w2788) -> ()  [unwired: 2 in, 2 out]
            n2216 = property on="Focus -" class="Bool (strict)"("Disabled"=w2788) -> ()  [unwired: 2 in, 2 out]
            n2217 = property on="Focus +" class="Bool (strict)"("Disabled"=w2788) -> ()  [unwired: 2 in, 2 out]
            n2218 = Number To Decimal String(number=w2778) -> (decimal integer string=w2814:string)  [unwired: 1 in]
            n2219 = property on="Focus -" class="Bool (strict)"() -> ("BoolText.Text"=w2789:string)  [unwired: 2 in, 2 out]
            n2220 = property on="Focus +" class="Bool (strict)"() -> ("BoolText.Text"=w2790:string)  [unwired: 2 in, 2 out]
            n2221 = case shown="True" "focusHome" {
              frame False {
              }
              frame True {
                n2222 = global read "Global_Telescopio.vi" "transactionId0MQ"() -> (w2878:u64)
                n2223 = Increment(x=w2878) -> (x+1=w2879:u64)
                n2224 = global write "Global_Telescopio.vi" "transactionId0MQ"(w2879) -> ()
                n2225 = call "Focus PUSH.vi"("action"="HOME" ("controller"), "clientTransactionId"=w2878) -> ()  [unwired: 9 in, 1 out]
              }
            }
            n2226 = case shown="True" "focusStop" {
              frame False {
              }
              frame True {
                n2227 = global read "Global_Telescopio.vi" "transactionId0MQ"() -> (w2831:u64)
                n2228 = Increment(x=w2831) -> (x+1=w2832:u64)
                n2229 = call "Focus PUSH.vi"("action"="HALT" ("controller"), "clientTransactionId"=w2831) -> ()  [unwired: 9 in, 1 out]
                n2230 = global write "Global_Telescopio.vi" "transactionId0MQ"(w2832) -> ()
              }
            }
            n2231 = case shown="False" "Focus -" {
              tunnel: w2814 -> [w2845 w2853]
              tunnel: w2789 -> [w2844 w2852]
              frame True {
                n2232 = case shown="\"OFF\"" w2844 {
                  tunnel: w2845 -> [_ w2850]
                  frame "ON", Default {
                  }
                  frame "OFF" {
                    n2233 = global read "Global_Telescopio.vi" "transactionId0MQ"() -> (w2847:u64)
                    n2234 = Concatenate Strings("FOCUSIN=" ("controller"), w2850) -> (w2849:string)
                    n2235 = Increment(x=w2847) -> (x+1=w2848:u64)
                    n2236 = call "Focus PUSH.vi"("action"=w2849, "clientTransactionId"=w2847) -> ()  [unwired: 9 in, 1 out]
                    n2237 = global write "Global_Telescopio.vi" "transactionId0MQ"(w2848) -> ()
                    n2238 = property on="Focus -" class="Bool (strict)"("BoolText.Text"="ON") -> ()  [unwired: 2 in, 2 out]
                  }
                }
              }
              frame False {
                n2239 = case shown="\"ON\"" w2852 {
                  tunnel: w2853 -> [_ _]
                  frame "ON" {
                    n2240 = global read "Global_Telescopio.vi" "transactionId0MQ"() -> (w2855:u64)
                    n2241 = property on="Focus -" class="Bool (strict)"("BoolText.Text"="OFF") -> ()  [unwired: 2 in, 2 out]
                    n2242 = Increment(x=w2855) -> (x+1=w2856:u64)
                    n2243 = global write "Global_Telescopio.vi" "transactionId0MQ"(w2856) -> ()
                    n2244 = call "Focus PUSH.vi"("action"="HALT" ("controller"), "clientTransactionId"=w2855) -> ()  [unwired: 9 in, 1 out]
                  }
                  frame "OFF", Default {
                  }
                }
              }
            }
            n2245 = case shown="True" "focusGo" {
              frame False {
              }
              frame True {
                n2246 = global read "Global_Telescopio.vi" "transactionId0MQ"() -> (w2872:u64)
                n2247 = Number To Decimal String(number="Setpoint") -> (decimal integer string=w2876:string)  [unwired: 1 in]
                n2248 = Concatenate Strings("MOVE=" ("controller"), w2876) -> (w2874:string)
                n2249 = Increment(x=w2872) -> (x+1=w2873:u64)
                n2250 = global write "Global_Telescopio.vi" "transactionId0MQ"(w2873) -> ()
                n2251 = call "Focus PUSH.vi"("action"=w2874, "clientTransactionId"=w2872) -> ()  [unwired: 9 in, 1 out]
              }
            }
            n2252 = case shown="False" "Focus +" {
              tunnel: w2814 -> [w2859 w2867]
              tunnel: w2790 -> [w2858 w2866]
              frame True {
                n2253 = case shown="\"OFF\"" w2858 {
                  tunnel: w2859 -> [w2864 _]
                  frame "OFF" {
                    n2254 = global read "Global_Telescopio.vi" "transactionId0MQ"() -> (w2860:u64)
                    n2255 = property on="Focus +" class="Bool (strict)"("BoolText.Text"="ON") -> ()  [unwired: 2 in, 2 out]
                    n2256 = Concatenate Strings("FOCUSOUT=" ("controller"), w2864) -> (w2863:string)
                    n2257 = Increment(x=w2860) -> (x+1=w2861:u64)
                    n2258 = call "Focus PUSH.vi"("action"=w2863, "clientTransactionId"=w2860) -> ()  [unwired: 9 in, 1 out]
                    n2259 = global write "Global_Telescopio.vi" "transactionId0MQ"(w2861) -> ()
                  }
                  frame "ON", Default {
                  }
                }
              }
              frame False {
                n2260 = case shown="\"ON\"" w2866 {
                  tunnel: w2867 -> [_ _]
                  frame "ON" {
                    n2261 = global read "Global_Telescopio.vi" "transactionId0MQ"() -> (w2868:u64)
                    n2262 = property on="Focus +" class="Bool (strict)"("BoolText.Text"="OFF") -> ()  [unwired: 2 in, 2 out]
                    n2263 = Increment(x=w2868) -> (x+1=w2869:u64)
                    n2264 = global write "Global_Telescopio.vi" "transactionId0MQ"(w2869) -> ()
                    n2265 = call "Focus PUSH.vi"("action"="HALT" ("controller"), "clientTransactionId"=w2868) -> ()  [unwired: 9 in, 1 out]
                  }
                  frame "OFF", Default {
                  }
                }
              }
            }
          }
          frame "ROTATOR" {
            # "MUDANÇA 22/6/11:\nValor default passou a ser carregado no início deste VI."
            n2266 = case shown="True" "Set Rotator Angle" {
              frame False {
              }
              frame True {
                # "MUDANÇA 22/6/11:\nIncluída a formatação\nda string"
                n2267 = call "Formata_Numeros.vi"("Formato ex-> 7.2"="7.2", "Valor num"="New Angle") -> ("resulting string"=w2892:string)
                "Rotator Angle" <- w2892
                n2268 = global write "Global_Telescopio.vi" "guide_ang"(w2892) -> ()
              }
            }
            n2269 = global write "Global_Telescopio.vi" "Flag-Rotator"(FALSE ("Flag-Rotator")) -> ()
            n2270 = local read "Default Angle"() -> (w2885:string)
            n2271 = global read "Global_Telescopio.vi" "rotator_def"() -> (w2886:string)
            n2272 = Not Equal?(x=w2886, y=w2885) -> (x != y?=w2884:bool)
            n2273 = case shown="True" "SetRotatorDefAngle" {
              tunnel: w2885 -> [_ w2890]
              frame False {
              }
              frame True {
                n2274 = local write "Rotator Angle"(w2890) -> ()
                n2275 = global write "Global_Telescopio.vi" "guide_ang"(w2890) -> ()
              }
            }
            n2276 = case shown="True" w2884 {
              tunnel: w2886 -> [_ w2889]
              frame False {
              }
              frame True {
                n2277 = local write "Rotator Angle"(w2889) -> ()
                n2278 = global write "Global_Telescopio.vi" "guide_ang"(w2889) -> ()
                "Default Angle" <- w2889
              }
            }
          }
          frame "DOME" {
            w2902 = u16 15 items=["Alarme", "Atencao", "Erro", "Ocupado", "Plataforma", "LCB", "Trapeira", "Paravento", "DomoRap", "DomoCW", "DomoCCW", "TBD", "Em movimento", "TrapRUN", "TrapFCH", "TrapABT"] ("NomeStatus")
            w2903 = u16 14 items=["Alarme", "Atencao", "Erro", "Ocupado", "Plataforma", "LCB", "Trapeira", "Paravento", "DomoRap", "DomoCW", "DomoCCW", "TBD", "Em movimento", "TrapRUN", "TrapFCH", "TrapABT"] ("NomeStatus")
            w2904 = u16 13 items=["Alarme", "Atencao", "Erro", "Ocupado", "Plataforma", "LCB", "Trapeira", "Paravento", "DomoRap", "DomoCW", "DomoCCW", "TBD", "Em movimento", "TrapRUN", "TrapFCH", "TrapABT"] ("NomeStatus")
            w2914 = u16 3 items=["Alarme", "Atencao", "Erro", "Ocupado", "TBD", "LCB", "Trapeira", "Paravento", "DomoRap", "DomoCW", "DomoCCW", "TBD", "Em movimento", "TBD"] ("NomeStatus")
            # "20250912)"
            # "20250912)"
            # "MUDANÇA:\nO CW CCW comandos enviados ao controlador\nde girar e parar, estão escondidos. 26-01-2022"
            n2279 = disable-structure shown="Disabled" {
              frame Disabled {
                w2919 = TRUE  # CUP unlock enable
                # "Checa travamento CUP"
                n2280 = global read "Global_Telescopio.vi" "CupStartPos"() -> (w2921:i16)
                n2281 = global read "Global_Telescopio.vi" "RevCupTO"() -> (w2920:u32)
                n2282 = call "Checa destino cupula.vi"("Target"=w2921) -> ("moverCup"=w2924:bool)  [unwired: 6 in, 2 out]
                n2283 = call "TickTimeout.vi"("msInicial"=w2920, "msTimeout"=u32 8000) -> ("msTick"=w2926:u32, "Timeout"=w2922:bool)  [unwired: 1 out]
                n2284 = Compound Arithmetic op=AND(invert w2924, w2922, w2919) -> (w2925:bool)
                n2285 = case shown="True" w2924 {
                  tunnel: w2926 -> [_ w2932]
                  frame False {
                  }
                  frame True {
                    n2286 = global write "Global_Telescopio.vi" "RevCupTO"(w2932) -> ()
                    n2287 = local write "StatDome"("Moving" ("Status")) -> ()
                  }
                }
                n2288 = case shown="True" w2925 {
                  tunnel: w2926 -> [_ w2928]
                  frame False {
                  }
                  frame True {
                    w2931 = u16 4 items=["ZERO", "AH", "DEC", "TUBO", "CUP"] ("Controlador")
                    n2289 = global write "Global_Telescopio.vi" "RevCupTO"(w2928) -> ()
                    n2290 = local write "StatDome"("Waiting" ("Status")) -> ()
                    n2291 = call "Monta Comando.vi"("Comando"="PARAR", "Dispositivo"="PROG", "Controlador"=w2931) -> ()  [unwired: 2 in, 5 out]
                  }
                }
              }
              frame Disabled {
                # "20240820"
                n2292 = global read "Global_Telescopio.vi" "RevCupTO"() -> (w2934:u32)
                n2293 = global read "Global_Telescopio.vi" "QtdEtiquetas"() -> (w2941:i16)
                n2294 = local read "DestCUP"() -> (w2940:i16)
                n2295 = Divide(x=w2941, y=2) -> (x/y=w2939:dbl)
                n2296 = call "TickTimeout.vi"("msInicial"=w2934, "msTimeout"=u32 3000) -> ("msTick"=w2937:u32, "Timeout"=w2936:bool)  [unwired: 1 out]
                n2297 = Subtract(x=w2940, y=w2939) -> (x-y=w2942:dbl)
                n2298 = Add(x=w2940, y=w2939) -> (x+y=w2943:dbl)
                n2299 = Greater?(x=w2943, y=w2941) -> (0:w2944:bool)
                n2300 = Select(t=w2942, s=w2944, f=w2943) -> (s? t:f=w2945:dbl)
                n2301 = case shown="True" w2936 {
                  tunnel: w2937 -> [_ w2952]
                  tunnel: w2945 -> [_ w2947]
                  frame False {
                  }
                  frame True {
                    w2951 = u16 4 items=["ZERO", "AH", "DEC", "TUBO", "CUP"] ("Controlador")
                    n2302 = To Word Integer(number=w2947) -> (16bit integer=w2946:i16)
                    n2303 = global write "Global_Telescopio.vi" "RevCupTO"(w2952) -> ()
                    n2304 = Number To Decimal String(number=w2946) -> (decimal integer string=w2949:string)  [unwired: 1 in]
                    n2305 = local write "StatDome"("Reverting" ("Status")) -> ()
                    n2306 = call "Monta Comando.vi"("Set Point"=w2949, "Comando"="MOVER" ("Dispositivo"), "Dispositivo"="DOMO", "Controlador"=w2951) -> ()  [unwired: 1 in, 5 out]
                  }
                }
              }
              frame Disabled {
                # "20240820"
                n2307 = global read "Global_Telescopio.vi" "RevCupTO"() -> (w2954:u32)
                n2308 = call "TickTimeout.vi"("msInicial"=w2954, "msTimeout"=u32 10000) -> ("msTick"=w2957:u32, "Timeout"=w2956:bool)  [unwired: 1 out]
                n2309 = case shown="True" w2956 {
                  tunnel: w2957 -> [_ w2958]
                  frame False {
                  }
                  frame True {
                    w2961 = u16 4 items=["ZERO", "AH", "DEC", "TUBO", "CUP"] ("Controlador")
                    n2310 = global write "Global_Telescopio.vi" "RevCupTO"(w2958) -> ()
                    n2311 = local write "StatDome"("Wait2s" ("Status")) -> ()
                    n2312 = call "Monta Comando.vi"("Comando"="PARAR", "Dispositivo"="PROG", "Controlador"=w2961) -> ()  [unwired: 2 in, 5 out]
                  }
                }
              }
              frame Disabled {
                n2313 = global read "Global_Telescopio.vi" "RevCupTO"() -> (w2963:u32)
